vi "ALTS-2015 Display Pass Fail Status.vi"(8 "error in (no error)":errorcluster, 10 "Test Result":string, 11 "Station Enum":T1) -> (0 "error out":errorcluster)   [LabVIEW 2013]
doc: "Copyright © 2005, Soliton Technologies.\nAll rights reserved."
uses:
  Controls/ALTS-2015 Station Cluster.ctl
  Controls/ALTS-2015 Digital Output Options.ctl
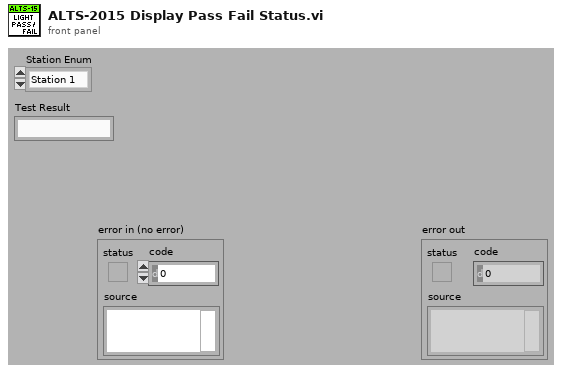
[diagram p1: front panel]
types:
  T1 = typedef "ALTS-2015 Station Cluster.ctl" = enum16{"Station 1", "Station 2", "Station 3", "Station 4"}
  T2 = typedef "ALTS-2015 Digital Output Options.ctl" = enum16{"Idle", "Test Running", "Pass", "Fail"}
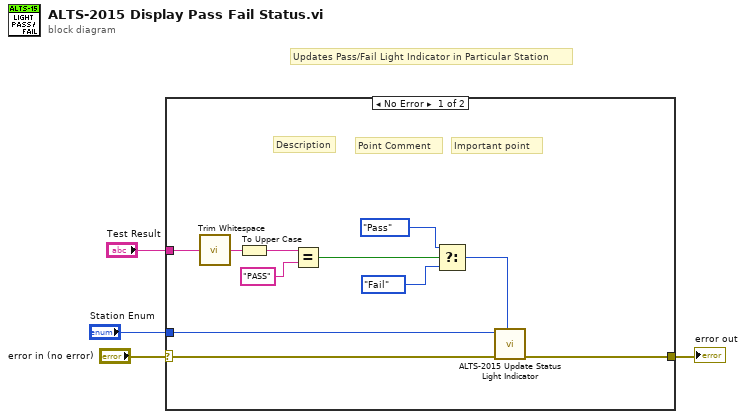
[diagram p0: block diagram]
diagram:
  # "Updates Pass/Fail Light Indicator in Particular Station"
  n1 = case shown="No Error" "error in (no error)" {
    selector: "error in (no error)" -> [w9 w16]
    tunnel: [w8 w16] -> w3
    tunnel: "Station Enum" -> [w7 _]
    tunnel: "Test Result" -> [w13 _]
    frame No Error {
      # "Point Comment"
      # "Important point"
      # "Description"
      n2 = call <vilib>:"Trim Whitespace.vi"("string"=w13) -> ("trimmed string"=w5:string)  [unwired: 1 in]
      n3 = To Upper Case(1:w5) -> (0:w15:string)
      n4 = Equal?(x=w15, y="PASS") -> (x = y?=w12:bool)
      n5 = Select(t=ALTS-2015_Digital_Output_Options."Pass" ("DO Options"), s=w12, f=ALTS-2015_Digital_Output_Options."Fail" ("DO Options")) -> (s? t:f=w6:T2)
      n6 = call "ALTS-2015 Update Status Light Indicator.vi"("DO Options"=w6, "error in"=w9, "Station Cluster"=w7) -> ("error out"=w8:errorcluster)  [unwired: 8 in]
    }
    frame Error {
    }
  }
  "error out" <- w3
